vi "send command to led controller.vi"(0 "Teensy Serial Port":refnum<visa-resource-name>, 1 "Command":T1(ring), 2 "lednumber":u8=1 min=1 max=2, 3 "stimulus1 value":u8, 4 "milliseconds to wait between write and read":u32=5, 5 "error in":errorcluster, 6 "num bytes to read":i32, 7 "file name":string, 8 "stimulus2 value":u8, 9 "output enabled":bool, 10 "logarithmic output?":bool, 11 "num bits per frame":u32, 12 "bytes to send":u8[](array[numeric])) -> (13 "command and response with time":string, 14 "teensy serial port out":refnum<visa-resource-name>, 15 "response":string, 17 "command sent":string, 18 "bytes read":u8[](array[numeric]), 19 "error out":errorcluster)   [LabVIEW 2013]
panel:
  # "/* Serial Commands\n * all commands on one line, terminate with \\n or \\r\n * R 1/2 filename - (Read) open file 1/2 for reading (use for experiment)\n * W filename - (Write) open file for writing\n * C - (Close) both files; done automatically at End of experiment\n * S 1/2 xxx - (Send) transfer xxx bytes from computer to file (specified by W) : xxx can be dec, hex (0x - zero x), or oct (leading 0 - zero)\n * F 1/2 xxx - (Fetch) transfer first xxx bytes from file to computer; if xxx is greater than number of bytes in file, remaining bytes will be 0 : xxx can be dec, hex (0x - zero x), or oct (leading 0 - zero)\n * S,F - xxx must be between 0 and 2^32-1 (maximum value of unsigned long); the conversion is handled by the c function strtoul, so xxx can be dec, hex (0x - zero x), or oct (leading 0 - zero)\n * O 1/2 x - (Output) 1/2 on (x > 0) or off (x == 0)\n *  note: opening a file for reading/writing automatically attempts to enable it\n * B - (Begin) experiment\n * E - (End) experiment\n * T xxx yyy - (sTimulus) set stimulus LED 1 to xxx and stimulus LED 2 to yyy\n * N xx - (Number) of bytes per frame; xx can be dec, hex, or oct, as ready by strtoi. xx must be > 0; unreasonably large values of xx will result in crashes\n * Y - (readY) - returns ready + details if ready to start experiment; returns error + details if not ready to start experiment\n * Q - (Quiet) - only respond to errors [default loud]\n * L - (Loud) - acknowledge all commands [default]\n * H - help - right, good luck with that guy\n* G 0/1 set logarithmic state (0 = linear, 1 = log)\n * I - Info - returns 5 long integers: A B C D E\\n\n *   A frame since experiment start if running; -999 if not running\n *   B time since experiment started in ms\n *   C position in file1 (note that experiment reads ahead)\n *   D position in file2 (note that experiment reads ahead)\n *   E number of bytes output to this point\n */"
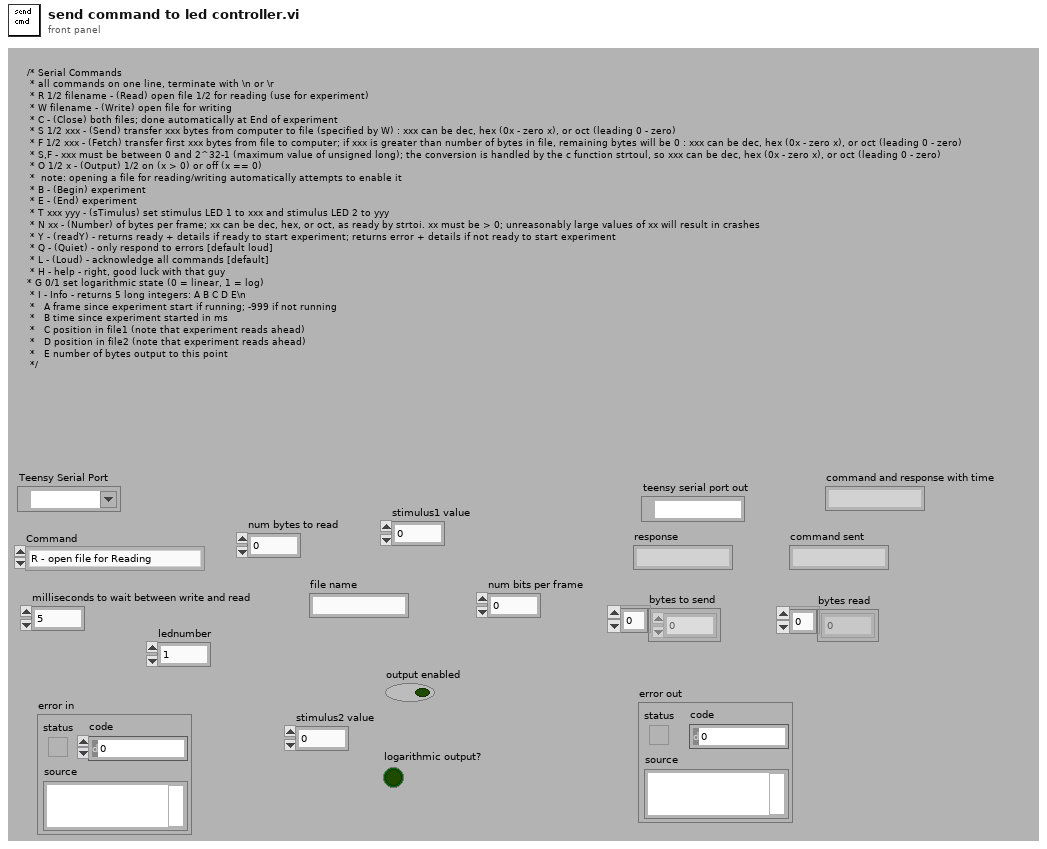
[diagram p1: front panel]
types:
  T1 = enum16{"R - open file for Reading", "W - open file for Writing", "S - send bytes", "F - fetch bytes", "B - begin experiment", "E - end experiment", "N - set number of bits per frame", "I - get info", "Q - Quiet (only error msgs)", "L - Loud (acknowledge all)", "T - set stimulus state", "Y - ready to start experiment", "H - useless Help message", "C - Close file", "O - enable/disable output", "G - set logarithmic output"}
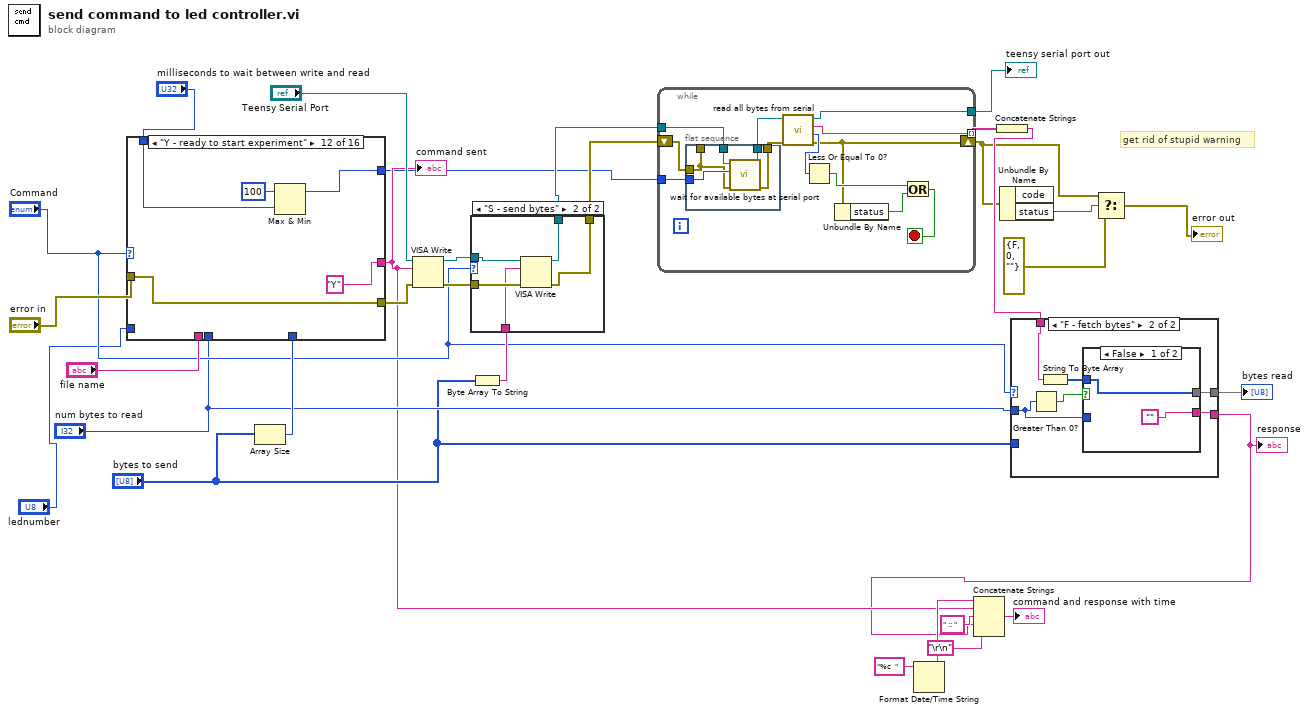
[diagram p0: block diagram]
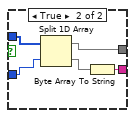
[diagram p3: hidden frame]
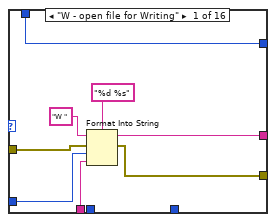
[diagram p5: hidden frame]
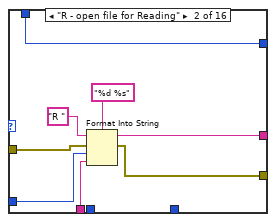
[diagram p6: hidden frame]
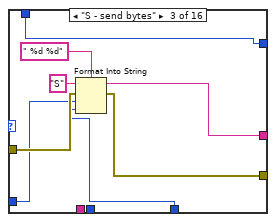
[diagram p7: hidden frame]
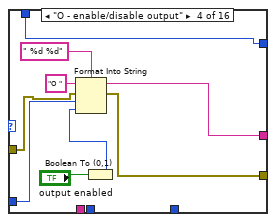
[diagram p8: hidden frame]
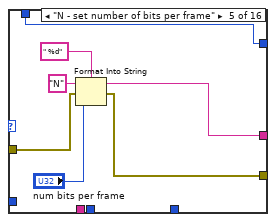
[diagram p9: hidden frame]
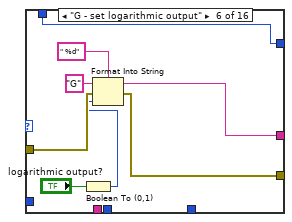
[diagram p10: hidden frame]
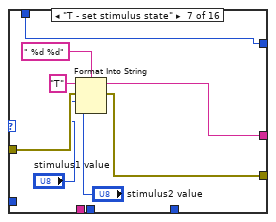
[diagram p11: hidden frame]
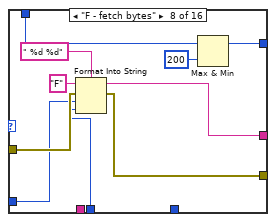
[diagram p12: hidden frame]
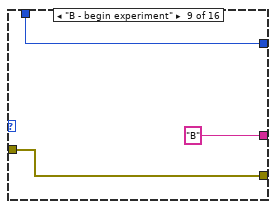
[diagram p13: hidden frame]
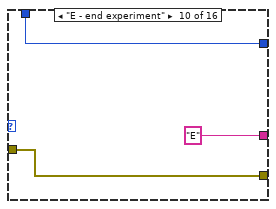
[diagram p14: hidden frame]
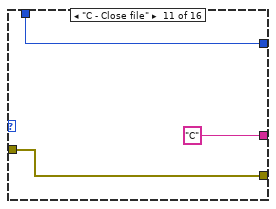
[diagram p15: hidden frame]
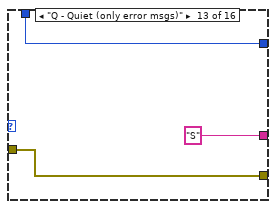
[diagram p16: hidden frame]
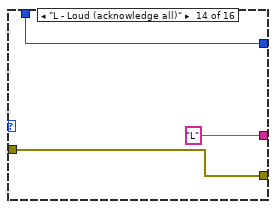
[diagram p17: hidden frame]
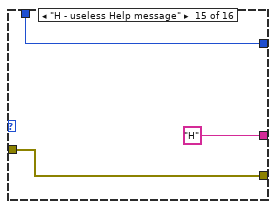
[diagram p18: hidden frame]
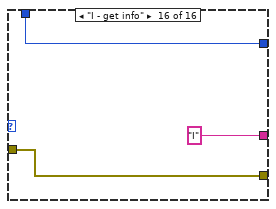
[diagram p19: hidden frame]
diagram:
  # "get rid of stupid warning"
  n1 = Array Size(array="bytes to send") -> (size(s)=w19:i32)
  n2 = case shown="\"Y - ready to start experiment\"" "Command" {
    tunnel: [w37 w45 w51 w60 w67 w75 w83 w93 "B" "E" "C" "Y" "S" "L" "H" "I"] -> w11
    tunnel: "error in" -> [w36 w44 w53 w62 w69 w77 w85 w95 w99 w102 w105 w111 w113 w117 w119 w122]
    tunnel: [w35 w43 w52 w61 w68 w76 w84 w94 w99 w102 w105 w111 w113 w117 w119 w122] -> w29
    tunnel: "file name" -> [w33 w42 _ _ _ _ _ _ _ _ _ _ _ _ _ _]
    tunnel: "num bytes to read" -> [_ _ _ _ _ _ _ w92 _ _ _ _ _ _ _ _]
    tunnel: w19 -> [_ _ w49 _ _ _ _ _ _ _ _ _ _ _ _ _]
    tunnel: "lednumber" -> [w34 w41 w50 w59 _ _ _ w91 _ _ _ _ _ _ _ _]
    tunnel: "milliseconds to wait between write and read" -> [w32 w40 w48 w56 w65 w74 w80 w90 w98 w101 w104 w109 w112 w115 w118 w121]
    tunnel: [w32 w40 w48 w56 w65 w74 w80 w89 w98 w101 w104 w108 w112 w115 w118 w121] -> w1
    frame "W - open file for Writing" {
      n3 = Format Into String(format string="%d %s", initial string="W ", error in=w36, w34, w33) -> (resulting string=w37:string, error out=w35:errorcluster)
    }
    frame "R - open file for Reading" {
      n4 = Format Into String(format string="%d %s", initial string="R ", error in=w44, w41, w42) -> (resulting string=w45:string, error out=w43:errorcluster)
    }
    frame "S - send bytes" {
      n5 = Format Into String(format string=" %d %d", initial string="S", error in=w53, w50, w49) -> (resulting string=w51:string, error out=w52:errorcluster)
    }
    frame "O - enable/disable output" {
      n6 = Boolean To (0,1)(Boolean="output enabled") -> (0, 1=w58:i16)
      n7 = Format Into String(format string=" %d %d", initial string="O ", error in=w62, w59, w58) -> (resulting string=w60:string, error out=w61:errorcluster)
    }
    frame "N - set number of bits per frame" {
      n8 = Format Into String(format string=" %d", initial string="N", error in=w69, "num bits per frame") -> (resulting string=w67:string, error out=w68:errorcluster)
    }
    frame "G - set logarithmic output" {
      n9 = Boolean To (0,1)(Boolean="logarithmic output?") -> (0, 1=w72:i16)
      n10 = Format Into String(format string=" %d", initial string="G", error in=w77, w72) -> (resulting string=w75:string, error out=w76:errorcluster)
    }
    frame "T - set stimulus state" {
      n11 = Format Into String(format string=" %d %d", initial string="T", error in=w85, "stimulus1 value", "stimulus2 value") -> (resulting string=w83:string, error out=w84:errorcluster)
    }
    frame "F - fetch bytes" {
      n12 = Format Into String(format string=" %d %d", initial string="F", error in=w95, w91, w92) -> (resulting string=w93:string, error out=w94:errorcluster)
      n13 = Max & Min(x=w90, y=u32 200) -> (max(x,y)=w89:u32)  [unwired: 1 out]
    }
    frame "B - begin experiment" {
    }
    frame "E - end experiment" {
    }
    frame "C - Close file" {
    }
    frame "Y - ready to start experiment" {
      n14 = Max & Min(x=u32 100, y=w109) -> (max(x,y)=w108:u32)  [unwired: 1 out]
    }
    frame "Q - Quiet (only error msgs)" {
    }
    frame "L - Loud (acknowledge all)" {
    }
    frame "H - useless Help message" {
    }
    frame "I - get info" {
    }
  }
  "command sent" <- w11
  n15 = VISA Write(VISA resource name="Teensy Serial Port", write buffer=w11, error in (no error)=w29) -> (VISA resource name out=w23:refnum<visa-resource-name>, error out=w24:errorcluster)  [unwired: 1 out]
  n16 = Byte Array To String(unsigned byte array="bytes to send") -> (string=w20:string)
  n17 = case shown="\"S - send bytes\"" "Command" {
    tunnel: w23 -> [w125 w130]
    tunnel: w24 -> [w124 w129]
    tunnel: [w125 w128] -> w22
    tunnel: [w124 w127] -> w21
    tunnel: w20 -> [_ w126]
    frame Default {
    }
    frame "S - send bytes" {
      n18 = VISA Write(VISA resource name=w130, write buffer=w126, error in (no error)=w129) -> (VISA resource name out=w128:refnum<visa-resource-name>, error out=w127:errorcluster)  [unwired: 1 out]
    }
  }
  n19 = while {
    tunnel: w22 -> [w133]
    tunnel: [w134] -> w28 mode=indexing
    shift-right: [w135] -> w6
    shift-left: w21 -> [w139]
    tunnel: w1 -> [w138]
    tunnel: [w137] -> w27
    stop <- w141 stop-if-true
    n20 = flat-sequence {
      tunnel: w139 -> [w146]
      tunnel: [w146] -> _
      tunnel: w138 -> [w147]
      tunnel: w133 -> [w145]
      tunnel: [w144] -> w132
      tunnel: [w143] -> w131
      frame #0 {
        n21 = call "wait for available bytes at serial port.vi"("error in (no error)"=w146, "ms to wait"=w147, "VISA resource name"=w145) -> ("error out"=w144:errorcluster, "VISA resource name 2"=w143:refnum<visa-resource-name>)  [unwired: 6 in, 1 out]
      }
    }
    n22 = call "read all bytes from serial.vi"("error in (no error)"=w132, "VISA resource name"=w131) -> ("error out"=w135:errorcluster, "nbytes read"=w136:i32, "concatenated string"=w134:string, "VISA resource name 2"=w137:refnum<visa-resource-name>)  [unwired: 6 in]
    n23 = Less Or Equal To 0?(x=w136) -> (x <= 0?=w140:bool)
    n24 = Unbundle By Name(w135) -> ("status"=w142:bool)
    n25 = Or(x=w140, y=w142) -> (x .or. y?=w141:bool)
  }
  "teensy serial port out" <- w27
  n26 = Format Date/Time String(time format string (%c)="%c  ") -> (date/time string=w12:string)  [unwired: 2 in]
  n27 = Concatenate Strings(w28) -> (w16:string)
  n28 = Unbundle By Name(w6) -> ("status"=w26:bool)  [unwired: 1 out]
  n29 = case shown="\"F - fetch bytes\"" "Command" {
    tunnel: "num bytes to read" -> [_ w151]
    tunnel: w16 -> [w148 w155]
    tunnel: [w149 w153] -> w15
    tunnel: "bytes to send" -> [w149 _]
    tunnel: [w148 w152] -> w9
    frame Default {
    }
    frame "F - fetch bytes" {
      n30 = Greater Than 0?(x=w151) -> (x > 0?=w150:bool)
      n31 = String To Byte Array(string=w155) -> (unsigned byte array=w154:u8[])
      n32 = case shown="False" w150 {
        tunnel: w154 -> [w157 w162]
        tunnel: w151 -> [_ w161]
        tunnel: [w157 w160] -> w153
        tunnel: ["" w158] -> w152
        frame False {
        }
        frame True {
          n33 = Split 1D Array(array=w162, index=w161) -> (first subarray=w160:u8[], second subarray=w159:u8[])
          n34 = Byte Array To String(unsigned byte array=w159) -> (string=w158:string)
        }
      }
    }
  }
  "response" <- w9
  "bytes read" <- w15
  n35 = Concatenate Strings(w12, w11, " :: " ("string"), w9, "\r\n") -> (→"command and response with time":string)
  n36 = Select(t=w6, s=w26, f=errorcluster {"status"=FALSE, "code"=0, "source"=""}) -> (s? t:f=→"error out":errorcluster)
